vi "Set_Names_ID_Projects.vi"(8 "error in (no error)":errorcluster, 11 "DB in":refnum<class "DB.lvclass">) -> (0 "error out":errorcluster, 3 "DB out":refnum<class "DB.lvclass">)   [LabVIEW 2015, in "DB.lvclass"]
uses:
  DB.lvclass
  DB.lvclass/DB.ctl
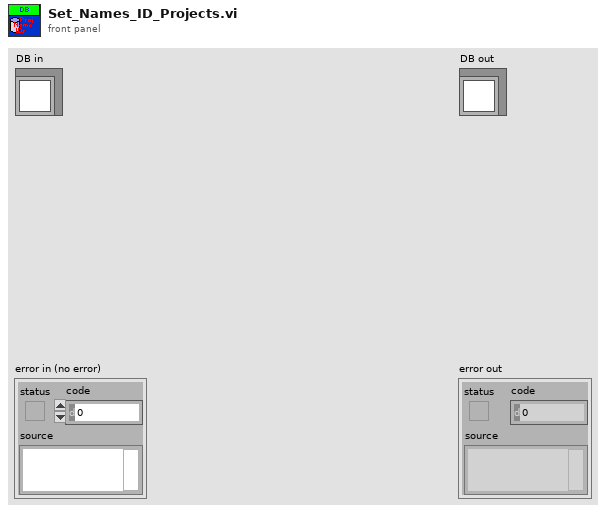
[diagram p1: front panel]
types:
  T1 = typedef "DB.lvclass/Def_fix_sql_param.ctl" = cluster{"Fix Project":bool, "Fix Sample":bool, "Fix Exp Date":bool, "Fix User":bool}
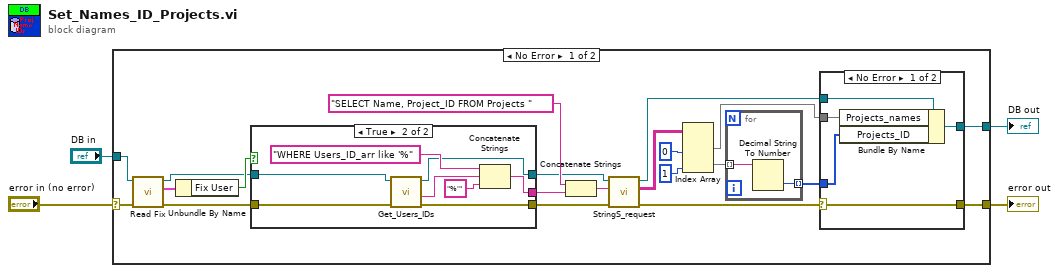
[diagram p0: block diagram]
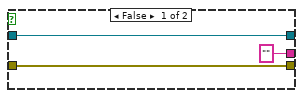
[diagram p2: hidden frame]
diagram:
  n1 = case shown="No Error" "error in (no error)" {
    selector: "error in (no error)" -> [w6 w47]
    tunnel: [w16 w47] -> w3
    tunnel: [w17 w46] -> w1
    tunnel: "DB in" -> [w7 w46]
    frame No Error {
      n2 = call "Read Fix.vi"("error in (no error)"=w6, "DB in"=w7) -> ("error out"=w10:errorcluster, "Fix"=w15:T1, "DB out"=w11:refnum<class "DB.lvclass">)  [unwired: 7 in]
      n3 = Unbundle By Name(w15) -> ("Fix User"=w14:bool)
      n4 = case shown="True" w14 {
        tunnel: ["" w35] -> w13
        tunnel: w11 -> [w28 w34]
        tunnel: [w28 w32] -> w8
        tunnel: w10 -> [w27 w31]
        tunnel: [w27 w30] -> w5
        frame False {
        }
        frame True {
          n5 = call "Get_Users_IDs.vi"("error in (no error)"=w31, "DB in"=w34) -> ("error out"=w30:errorcluster, "Project_ID_arr"=w33:string, "DB out"=w32:refnum<class "DB.lvclass">)  [unwired: 6 in, 1 out]
          n6 = Concatenate Strings("WHERE Users_ID_arr like '%", w33, "%'" ("string")) -> (w35:string)
        }
      }
      n7 = Concatenate Strings("SELECT Name, Project_ID FROM Projects " ("SQL"), w13) -> (w9:string)
      n8 = call-dynamic "StringS_request.vi"("error in (no error)"=w5, "SQL request"=w9, "DB in"=w8) -> ("error out"=w23:errorcluster, "Result Set"=w21:string[][], "DB out"=w25:refnum<class "DB.lvclass">)  [unwired: 5 in, 1 out]
      n9 = Index Array(array=w21, index (col) #1=0 ("disabled index (col)"), index (col) #2=1 ("index (col)")) -> (element #1=w24:string[], element #2=w20:string[])  [unwired: 2 in]
      n10 = for {
        tunnel: w20 -> [w45] mode=indexing
        tunnel: [w44] -> w22 mode=indexing
        n11 = Decimal String To Number(string=w45) -> (number=w44:i32)  [unwired: 2 in, 1 out]
      }
      n12 = case shown="No Error" w23 {
        selector: w23 -> [w37 w42]
        tunnel: w25 -> [w41 w43]
        tunnel: [w40 w43] -> w17
        tunnel: w22 -> [w39 _]
        tunnel: w24 -> [w38 _]
        tunnel: [w37 w42] -> w16
        frame No Error {
          n13 = Bundle By Name(cluster=w41, "Projects_names"=w38, "Projects_ID"=w39) -> (w40:refnum<class "DB.lvclass">)
        }
        frame Error {
        }
      }
    }
    frame Error {
    }
  }
  "error out" <- w3
  "DB out" <- w1
